vi "NumberCaseStructure.vi"() -> ()   [LabVIEW 2019]
panel:
  in  "month":u8
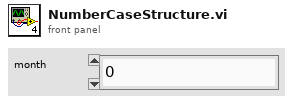
[diagram p1: front panel]
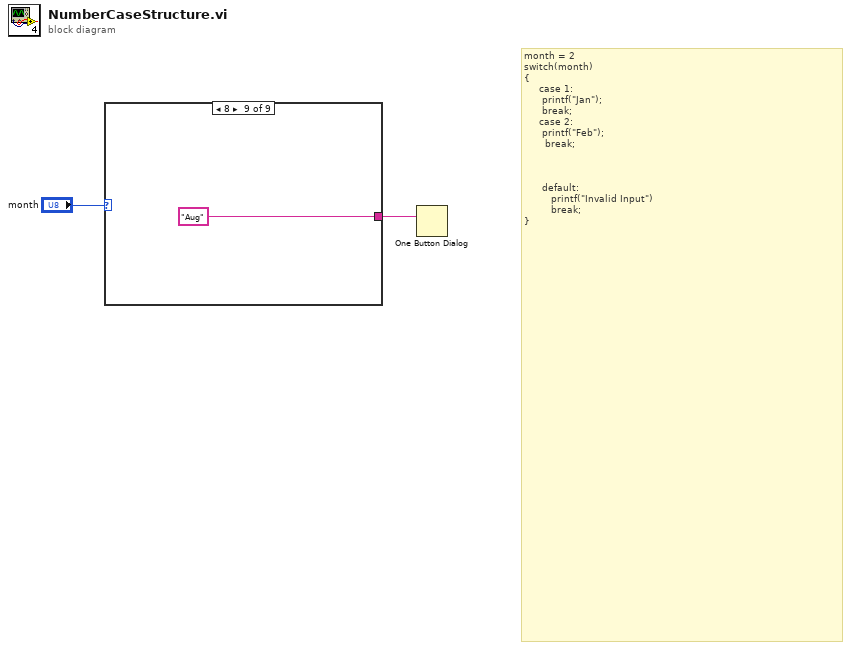
[diagram p0: block diagram]
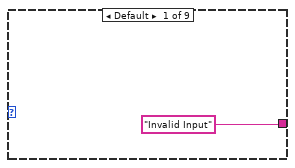
[diagram p2: hidden frame]
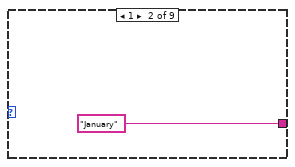
[diagram p3: hidden frame]
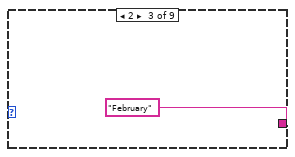
[diagram p4: hidden frame]
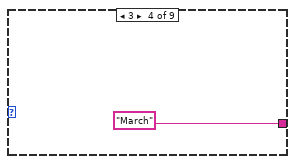
[diagram p5: hidden frame]
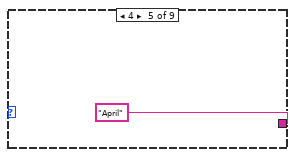
[diagram p6: hidden frame]
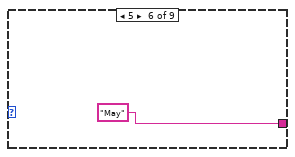
[diagram p7: hidden frame]
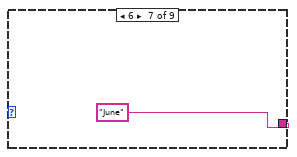
[diagram p8: hidden frame]
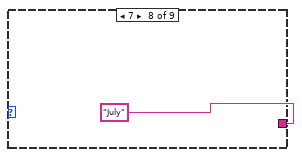
[diagram p9: hidden frame]
diagram:
  # "month = 2\nswitch(month)\n{\n     case 1:\n      printf(\"Jan\");\n      break;\n     case 2:\n      printf(\"Feb\");\n       break;\n     \n\n      \n      default:\n         printf(\"Invalid Input\")\n         break;\n}"
  n1 = case shown="8" "month" {
    tunnel: ["Invalid Input" ("message") "January" ("message") "February" ("message") "March" ("message") "April" ("message") "May" ("message") "June" ("message") "July" ("message") "Aug" ("message")] -> w1
    frame Default {
    }
    frame 1 {
    }
    frame 2 {
    }
    frame 3 {
    }
    frame 4 {
    }
    frame 5 {
    }
    frame 6 {
    }
    frame 7 {
    }
    frame 8 {
    }
  }
  n2 = One Button Dialog(message=w1) -> ()  [unwired: 1 in, 1 out]
